vi "build_graph-single_axis.vi"(8 "error in (no error)":errorcluster, 10 "y_axis":dbl[][](array[numeric]), 11 "x_axis":dbl[](array[numeric])) -> (0 "error out":errorcluster, 4 "graph_data":cluster{dbl[], dbl[]}[](array[cluster]), 6 "scale_ranges":T1)   [LabVIEW 2015, in "lv-graph.lvlib"]
uses:
  lv-graph.lvlib
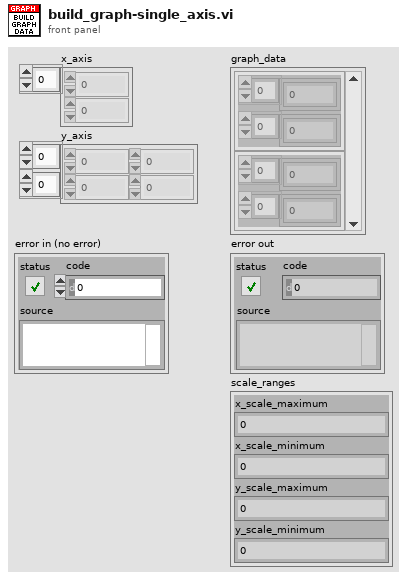
[diagram p1: front panel]
types:
  T1 = cluster{"x_scale_maximum":dbl, "x_scale_minimum":dbl, "y_scale_maximum":dbl, "y_scale_minimum":dbl}
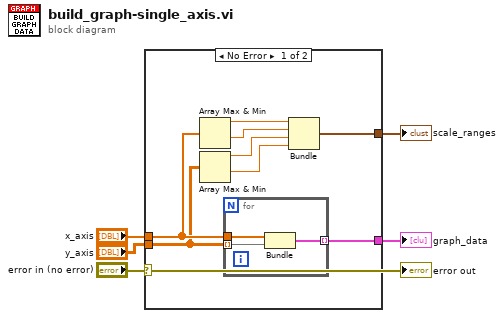
[diagram p0: block diagram]
diagram:
  n1 = case shown="No Error" "error in (no error)" {
    tunnel: [w13 _] -> w5
    tunnel: "y_axis" -> [w11 _]
    tunnel: "x_axis" -> [w12 _]
    tunnel: [w7 _] -> w2
    frame No Error {
      n2 = Array Max & Min(array=w12) -> (max value=w10:dbl, min value=w6:dbl)  [unwired: 2 out]
      n3 = Array Max & Min(array=w11) -> (max value=w9:dbl, min value=w8:dbl)  [unwired: 2 out]
      n4 = for {
        tunnel: w12 -> [w15]
        tunnel: w11 -> [w16] mode=indexing
        tunnel: [w14] -> w13 mode=indexing
        n5 = Bundle("x_axis"=w15, "y_axis"=w16) -> (w14:cluster{"x_axis":dbl[], "y_axis":dbl[]})  [unwired: 1 in]
      }
      n6 = Bundle(w10, w6, w9, w8) -> (w7:cluster{dbl, dbl, dbl, dbl})  [unwired: 1 in]
    }
    frame Error {
    }
  }
  "graph_data" <- w5
  "scale_ranges" <- w2
  "error out" <- "error in (no error)"
